vi "setCommandValveAngle00.vi"(1 "error in (no error)":errorcluster, 2 "angle(deg)":dbl) -> (0 "error out":errorcluster)   [LabVIEW 2011]
panel:
  out "concatenated string":string
  out "VISA resource name out":refnum<visa-resource-name>
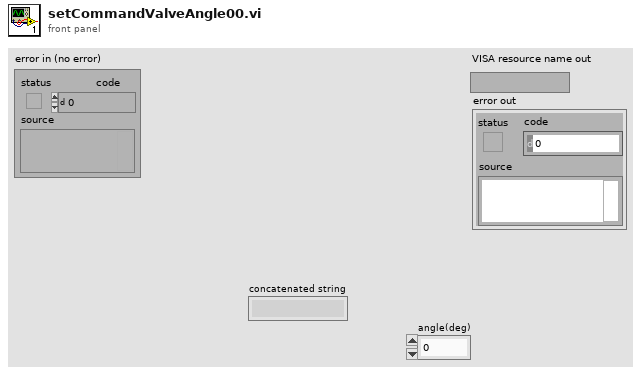
[diagram p1: front panel]
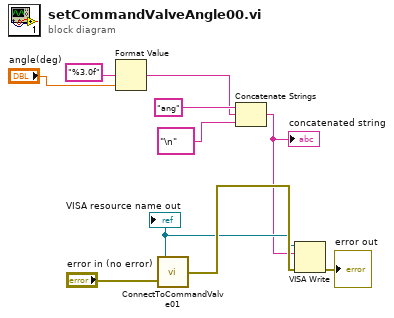
[diagram p0: block diagram]
diagram:
  n1 = Format Value(format string="%3.0f", value (0)="angle(deg)") -> (output string=w1:string)  [unwired: 1 in]
  n2 = call "ConnectToCommandValve01.vi"("error in (no error)"="error in (no error)") -> ("error out"=w9:errorcluster, "VISA resource name out"=w8:refnum<visa-resource-name>)
  "VISA resource name out" <- w8
  n3 = Concatenate Strings("ang" ("string to write"), w1, "\n") -> (w5:string)
  "concatenated string" <- w5
  n4 = VISA Write(VISA resource name=w8, write buffer=w5, error in (no error)=w9) -> (error out=→"error out":errorcluster)  [unwired: 2 out]
